vi "DeleteParametricWaveform.vi"(1 "Waveform Name":string, 3 "error in (no error)":errorcluster, 4 "Selection":u16(ring)=1 items=["All Parametric Waveforms", "Specific Waveform"], 5 "VISA resource name":refnum<visa-resource-name>) -> (0 "error out":errorcluster, 2 "VISA resource name out":refnum<visa-resource-name>)   [LabVIEW 2020, in "Active Technologies AWG3000.lvlib"]
uses:
  Active Technologies AWG3000.lvlib
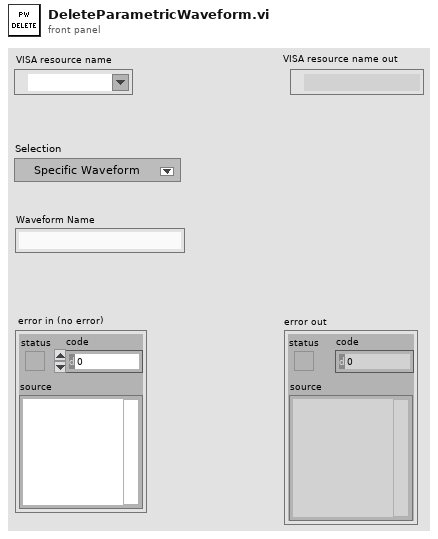
[diagram p1: front panel]
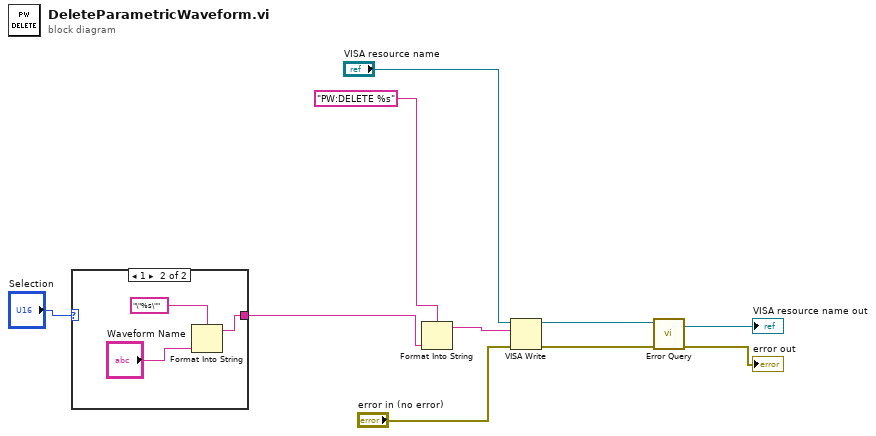
[diagram p0: block diagram]
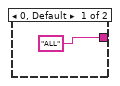
[diagram p2: hidden frame]
diagram:
  n1 = case shown="1" "Selection" {
    tunnel: ["ALL" ("write buffer") w12] -> w1
    frame 0, Default {
    }
    frame 1 {
      n2 = Format Into String(format string="\"%s\"" ("write buffer"), "Waveform Name") -> (resulting string=w12:string)  [unwired: 2 in, 1 out]
    }
  }
  n3 = Format Into String(format string="PW:DELETE %s" ("write buffer"), w1) -> (resulting string=w4:string)  [unwired: 2 in, 1 out]
  n4 = VISA Write(VISA resource name="VISA resource name", write buffer=w4, error in (no error)="error in (no error)") -> (VISA resource name out=w8:refnum<visa-resource-name>, error out=w7:errorcluster)  [unwired: 1 out]
  n5 = call "Error Query.vi"("error in (no error)"=w7, "VISA resource name"=w8) -> ("error out"=→"error out":errorcluster, "VISA resource name out"=→"VISA resource name out":refnum<visa-resource-name>)  [unwired: 6 in, 2 out]
